vi "get_AnalysisInfo.vi"(8 "error in (no error)":errorcluster, 11 "Analysis in":refnum<class "Analysis.lvclass">) -> (0 "error out":errorcluster, 2 "AnalysisInfo out":string, 3 "Analysis out":refnum<class "Analysis.lvclass">)   [LabVIEW 2017, in "Analysis.lvclass"]
doc: "returns a string with the analysis info\nRunID\nAnalysisID\nAnalysisName\nAnalysisType\nAnalysisDate\nAnalysisTime\nAnalysisTimeStamp"
uses:
  Analysis.lvclass
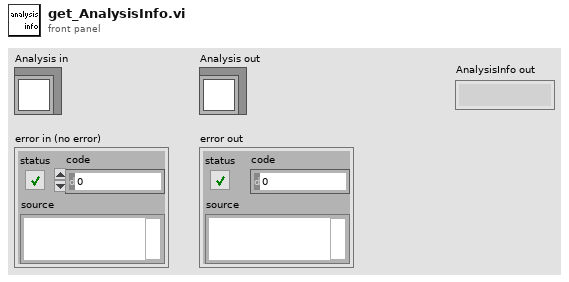
[diagram p1: front panel]
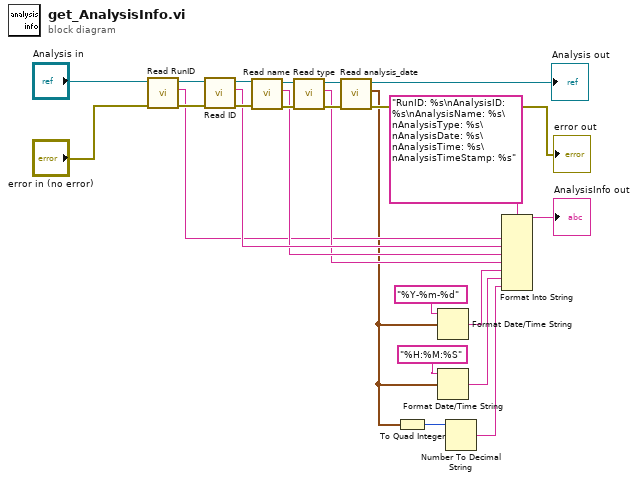
[diagram p0: block diagram]
diagram:
  n1 = call-dynamic "Read RunID.vi"("error in (no error)"="error in (no error)", "Analysis in"="Analysis in") -> ("error out"=w11:errorcluster, "RunID"=w8:string, "Analysis out"=w12:refnum<class "Analysis.lvclass">)  [unwired: 7 in]
  n2 = call-dynamic "Read ID.vi"("error in (no error)"=w11, "Analysis in"=w12) -> ("error out"=w19:errorcluster, "ID"=w16:string, "Analysis out"=w18:refnum<class "Analysis.lvclass">)  [unwired: 7 in]
  n3 = call-dynamic "Read name.vi"("error in (no error)"=w19, "Analysis in"=w18) -> ("error out"=w21:errorcluster, "name"=w15:string, "Analysis out"=w20:refnum<class "Analysis.lvclass">)  [unwired: 7 in]
  n4 = call-dynamic "Read type.vi"("error in (no error)"=w21, "Analysis in"=w20) -> ("error out"=w23:errorcluster, "type"=w14:string, "Analysis out"=w22:refnum<class "Analysis.lvclass">)  [unwired: 7 in]
  n5 = call-dynamic "Read analysis_date.vi"("error in (no error)"=w23, "Analysis in"=w22) -> ("error out"=→"error out":errorcluster, "analysis date"=w3:timestamp, "Analysis out"=→"Analysis out":refnum<class "Analysis.lvclass">)  [unwired: 7 in]
  n6 = To Quad Integer(1:w3) -> (0:w2:i64)
  n7 = Format Date/Time String(time format string (%c)="%Y-%m-%d", seconds (now)=w3) -> (date/time string=w6:string)  [unwired: 1 in]
  n8 = Format Date/Time String(time format string (%c)="%H:%M:%S", seconds (now)=w3) -> (date/time string=w4:string)  [unwired: 1 in]
  n9 = Number To Decimal String(number=w2) -> (decimal integer string=w1:string)  [unwired: 1 in]
  n10 = Format Into String(format string="RunID: %s\nAnalysisID: %s\nAnalysisName: %s\nAnalysisType: %s\nAnalysisDate: %s\nAnalysisTime: %s\nAnalysisTimeStamp: %s", w8, w16, w15, w14, w6, w4, w1) -> (resulting string=→"AnalysisInfo out":string)  [unwired: 2 in, 1 out]
